vi "Sum Vector Elements.vi"(1 "A x B":T1) -> (0 "Numeric":dbl)   [LabVIEW 2014]
uses:
  <vilib>/Analysis/Matrix/Datatypes/RealMatrix.ctl
  <vilib>/Analysis/Matrix/NI_Matrix.lvlib
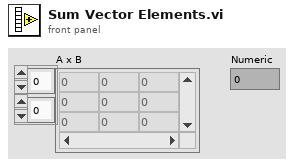
[diagram p1: front panel]
types:
  T1 = typedef "NI_Matrix.lvlib/RealMatrix.ctl" = dbl[][]
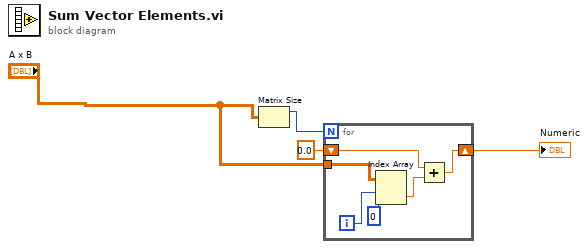
[diagram p0: block diagram]
diagram:
  n1 = Matrix Size(0:"A x B") -> (1:w2:i32)  [unwired: 1 out]
  n2 = for {
    N: w2 -> [_]
    shift-right: [w6] -> w3
    shift-left: 0.0 -> [w5]
    tunnel: "A x B" -> [w8]
    i -> [w10]
    n3 = Index Array(array=w8, index (row)=w10, index (col)=0) -> (element=w7:dbl)
    n4 = Add(x=w5, y=w7) -> (x+y=w6:dbl)
  }
  "Numeric" <- w3
